vi "Self-Test.vi"(8 "error in (no error)":errorcluster, 11 "VISA resource name":refnum<visa-resource-name>) -> (0 "error out":errorcluster, 1 "Self-Test Result Message":string, 2 "Self-Test Result Code":i32, 3 "VISA resource name out":refnum<visa-resource-name>)   [LabVIEW 2018, in "Keithley 3706.lvlib"]
uses:
  <instrlib>/Keithley 3706/Keithley 3706.lvlib
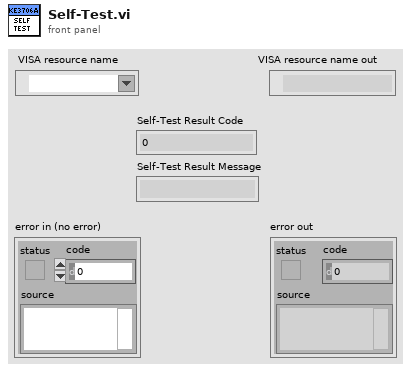
[diagram p1: front panel]
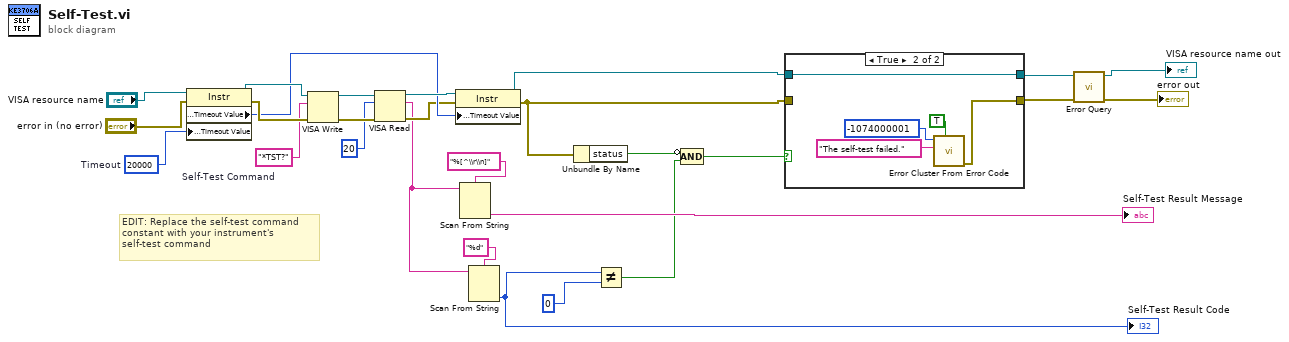
[diagram p0: block diagram]
diagram:
  w22 = "*TST?"  # Self-Test Command
  w25 = u32 20000  # Timeout
  # "EDIT: Replace the self-test command\nconstant with your instrument's\nself-test command"
  n1 = property class="Instr"(reference="VISA resource name", error in="error in (no error)", "General Settings:Timeout Value"=w25) -> (reference out=w24:refnum<visa-resource-name>, error out=w23:errorcluster, "General Settings:Timeout Value"=w17:u32)
  n2 = VISA Write(VISA resource name=w24, write buffer=w22, error in (no error)=w23) -> (VISA resource name out=w21:refnum<visa-resource-name>, error out=w20:errorcluster)  [unwired: 1 out]
  n3 = VISA Read(VISA resource name=w21, byte count=u32 20 ("byte count (20)"), error in (no error)=w20) -> (VISA resource name out=w18:refnum<visa-resource-name>, read buffer=w14:string, error out=w16:errorcluster)  [unwired: 1 out]
  n4 = property class="Instr"(reference=w18, error in=w16, "General Settings:Timeout Value"=w17) -> (reference out=w7:refnum<visa-resource-name>, error out=w6:errorcluster)
  n5 = Scan From String(format string="%[^\\r\\n]" ("Format String"), input string=w14) -> (output 1=→"Self-Test Result Message":string)  [unwired: 3 in, 3 out]
  n6 = Scan From String(format string="%d", input string=w14) -> (output 1=w11:i32)  [unwired: 3 in, 3 out]
  "Self-Test Result Code" <- w11
  n7 = Unbundle By Name(w6) -> ("status"=w9:bool)
  n8 = Not Equal?(x=w11, y=0) -> (x != y?=w8:bool)
  n9 = Compound Arithmetic op=AND(invert w9, w8) -> (w5:bool)
  n10 = case shown="True" w5 {
    tunnel: w7 -> [w29 w30]
    tunnel: w6 -> [w28 _]
    tunnel: [w29 w30] -> w4
    tunnel: [w28 w31] -> w3
    frame False {
    }
    frame True {
      n11 = call <vilib>:"Error Cluster From Error Code.vi"("show call chain? (False)"=TRUE, "error message (\"\")"="The self-test failed." ("Source (VI Name)"), "error code (0)"=-1074000001 ("Code")) -> ("error out"=w31:errorcluster)  [unwired: 6 in]
    }
  }
  n12 = call <instrlib>:"Error Query.vi"("error in (no error)"=w3, "VISA resource name"=w4) -> ("error out"=→"error out":errorcluster, "VISA resource name output"=→"VISA resource name out":refnum<visa-resource-name>)  [unwired: 6 in, 2 out]
